vi "ExSubtract2DataFiles.vi"() -> ()   [LabVIEW 2010]
panel:
  in  "Output File Type":u32=67371008
  in  "Output File Name":path
  in  "Input File 2 Type":u32=67371008
  in  "Input File 2 Operation":u32=6
  in  "Input File 1 Name":path
  in  "Input File 2 Name":path
  in  "Input File 1 Operation":u32=6
  in  "Input File 1 Type":u32=67371008
  out "error out":errorcluster
  in  "error in (no error)":errorcluster
  # "ExSubtract2DataFiles.vi\nThis VI will open the both input files, subtract File 2 from File 1\nand save the result to the output file. \nNote that the full path names must be provided for both input\nfiles and the output file."
  # "TIF   = 67174400\n  SPE = 67371008\n  PMI  = 67436544"
  # "6 = Read Only"
  # "TIF   = 67174400\n  SPE = 67371008\n  PMI  = 67436544"
  # "6 = Read Only"
  # "TIF   = 67174400\n  SPE = 67371008\n  PMI  = 67436544"
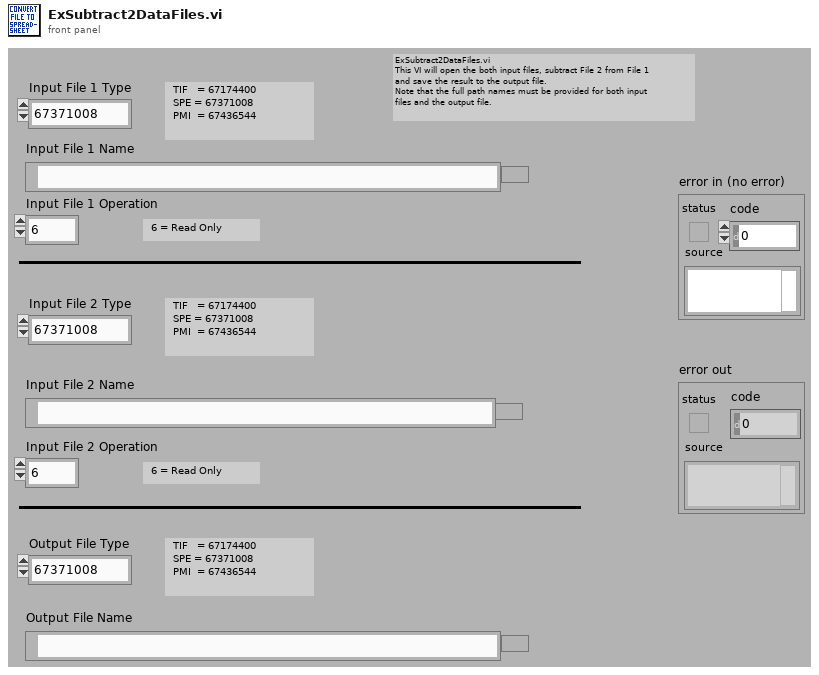
[diagram p1: front panel]
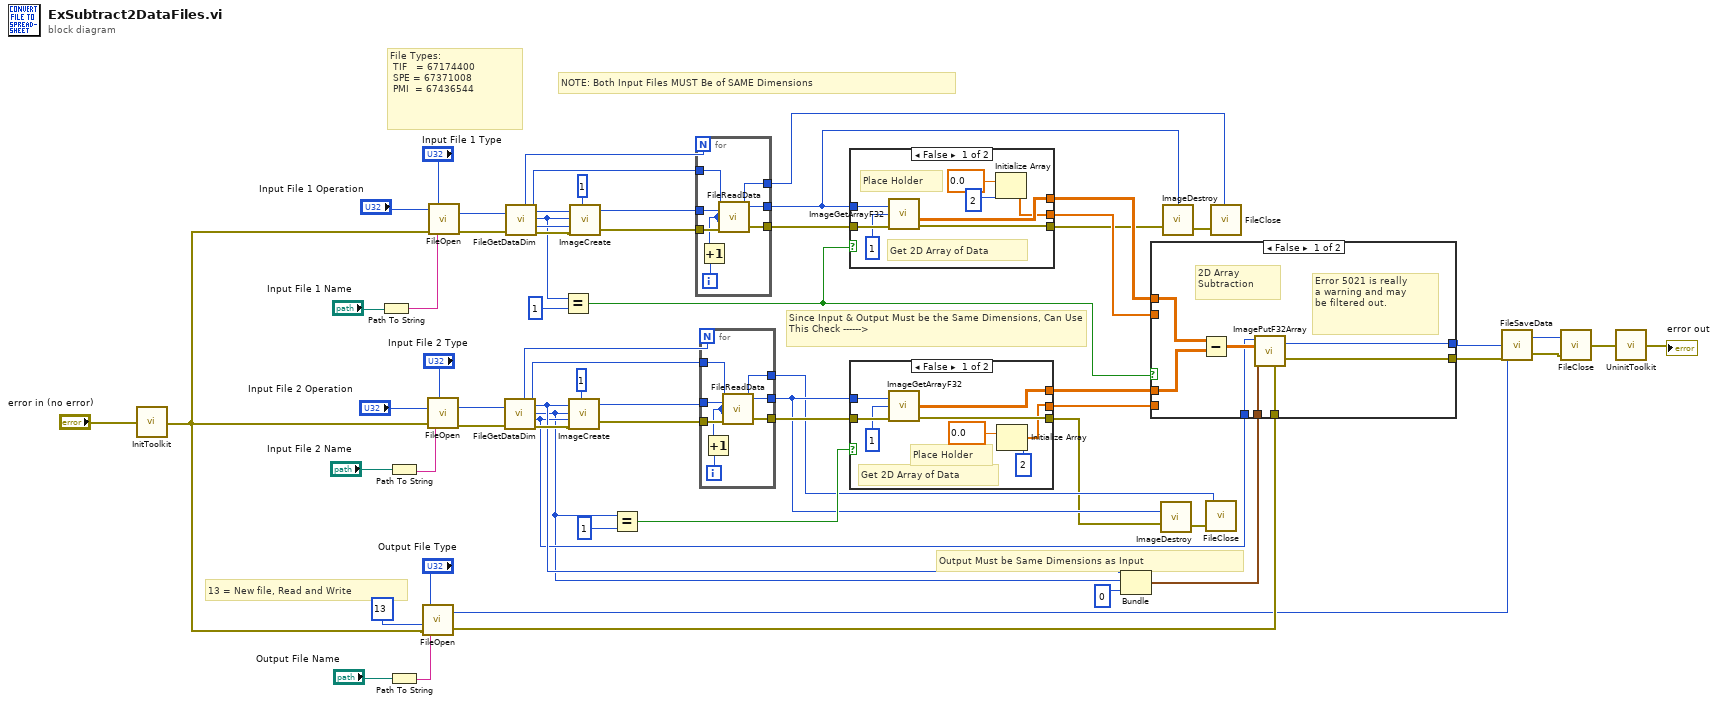
[diagram p0: block diagram]
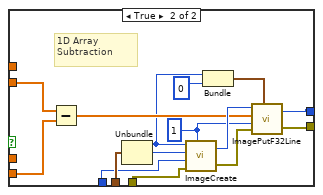
[diagram p2: hidden frame]
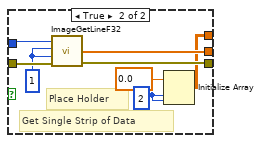
[diagram p3: hidden frame]
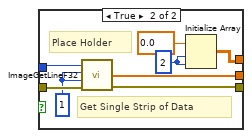
[diagram p4: hidden frame]
diagram:
  # "Since Input & Output Must be the Same Dimensions, Can Use This Check ------>"
  # "NOTE: Both Input Files MUST Be of SAME Dimensions"
  # "Output Must be Same Dimensions as Input"
  # "13 = New file, Read and Write"
  # "File Types:\n TIF   = 67174400\n SPE = 67371008\n PMI  = 67436544"
  n1 = call <userlib>:"InitToolkit.vi"("error in"="error in (no error)") -> ("error out"=w1:errorcluster)
  n2 = Path To String(path="Input File 1 Name") -> (string=w48:string)
  n3 = Path To String(path="Input File 2 Name") -> (string=w37:string)
  n4 = Path To String(path="Output File Name") -> (string=w27:string)
  n5 = call <userlib>:"FileOpen.vi"("error in"=w1, "File Operations"=13, "FileName"=w27, "File Type"="Output File Type") -> ("error out"=w8:errorcluster, "File Handle"=w3:u32)
  n6 = call <userlib>:"FileOpen.vi"("error in"=w1, "File Operations"="Input File 2 Operation", "FileName"=w37, "File Type"="Input File 2 Type") -> ("error out"=w44:errorcluster, "File Handle"=w43:u32)
  n7 = call <userlib>:"FileOpen.vi"("error in"=w1, "File Operations"="Input File 1 Operation", "FileName"=w48, "File Type"="Input File 1 Type") -> ("error out"=w62:errorcluster, "File Handle"=w61:u32)
  n8 = call <userlib>:"FileGetDataDim.vi"("File Handle"=w43, "error in"=w44) -> ("Number of Frames"=w35:u32, "Data Type"=w12:u32, "File Handle"=w34:u32, "X dim"=w13:u32, "Y dim"=w11:u32, "error out"=w42:errorcluster)
  n9 = call <userlib>:"FileGetDataDim.vi"("File Handle"=w61, "error in"=w62) -> ("Number of Frames"=w59:u32, "Data Type"=w26:u32, "File Handle"=w57:u32, "X dim"=w49:u32, "Y dim"=w25:u32, "error out"=w60:errorcluster)
  n10 = Equal?(x=w25, y=1) -> (x = y?=w20:bool)
  n11 = call <userlib>:"ImageCreate.vi"("X dimension"=w13, "Y dimension"=w11, "Data Type"=w12, "error in"=w42, "Number Of Frames"=1) -> ("Image Handle"=w33:u32, "error out"=w32:errorcluster)
  n12 = call <userlib>:"ImageCreate.vi"("X dimension"=w49, "Y dimension"=w25, "Data Type"=w26, "error in"=w60, "Number Of Frames"=1) -> ("Image Handle"=w56:u32, "error out"=w47:errorcluster)
  n13 = Equal?(x=w11, y=1) -> (x = y?=w30:bool)
  n14 = for {
    N: w59 -> [_]
    tunnel: w47 -> [w72]
    tunnel: w57 -> [w71]
    tunnel: w56 -> [w70]
    tunnel: [w65] -> w45
    tunnel: [w67] -> w55
    tunnel: [w66] -> w46
    i -> [w69]
    n15 = Increment(x=w69) -> (x+1=w68:i32)
    n16 = call <userlib>:"FileReadData.vi"("File Handle"=w71, "Start Frame"=w68, "End Frame"=w68, "error in"=w72, "Image Handle"=w70) -> ("File Handle"=w67:u32, "Image Handle"=w66:u32, "error out"=w65:errorcluster)
  }
  n17 = for {
    N: w35 -> [_]
    tunnel: w32 -> [w80]
    tunnel: w34 -> [w79]
    tunnel: w33 -> [w78]
    tunnel: [w73] -> w31
    tunnel: [w75] -> w21
    tunnel: [w74] -> w22
    i -> [w77]
    n18 = Increment(x=w77) -> (x+1=w76:i32)
    n19 = call <userlib>:"FileReadData.vi"("File Handle"=w79, "Start Frame"=w76, "End Frame"=w76, "error in"=w80, "Image Handle"=w78) -> ("File Handle"=w75:u32, "Image Handle"=w74:u32, "error out"=w73:errorcluster)
  }
  n20 = case shown="False" w20 {
    tunnel: w45 -> [w88 w95]
    tunnel: [w86 w96] -> w14
    tunnel: w46 -> [w85 w94]
    tunnel: [w81 w92] -> w17
    tunnel: [w84 w90] -> w19
    frame False {
      # "Place Holder"
      # "Get 2D Array of Data"
      n21 = call <userlib>:"ImageGetArrayF32.vi"("error in"=w88, "Z position"=1, "Image Handle"=w85) -> ("error out"=w86:errorcluster, "Array Float 32"=w84:sgl[][])  [unwired: 1 out]
      n22 = Initialize Array(sgl 0.0, 2) -> (w81:sgl[])
    }
    frame True {
      w89 = 2
      w93 = 1
      # "Place Holder"
      # "Get Single Strip of Data"
      n23 = call <userlib>:"ImageGetLineF32.vi"("error in"=w95, "Z Position"=w93, "Y Position"=w93, "Data Handle"=w94) -> ("error out"=w96:errorcluster, "Array F32"=w92:sgl[])  [unwired: 1 out]
      n24 = Initialize Array(sgl 0.0, w89, w89) -> (w90:sgl[][])
    }
  }
  n25 = case shown="False" w30 {
    tunnel: w31 -> [w104 w111]
    tunnel: [w102 w112] -> w15
    tunnel: w22 -> [w101 w110]
    tunnel: [w97 w108] -> w16
    tunnel: [w100 w105] -> w18
    frame False {
      # "Place Holder"
      # "Get 2D Array of Data"
      n26 = call <userlib>:"ImageGetArrayF32.vi"("error in"=w104, "Z position"=1, "Image Handle"=w101) -> ("error out"=w102:errorcluster, "Array Float 32"=w100:sgl[][])  [unwired: 1 out]
      n27 = Initialize Array(sgl 0.0, 2) -> (w97:sgl[])
    }
    frame True {
      w106 = 2
      w109 = 1
      # "Place Holder"
      # "Get Single Strip of Data"
      n28 = call <userlib>:"ImageGetLineF32.vi"("error in"=w111, "Z Position"=w109, "Y Position"=w109, "Data Handle"=w110) -> ("error out"=w112:errorcluster, "Array F32"=w108:sgl[])  [unwired: 1 out]
      n29 = Initialize Array(sgl 0.0, w106, w106) -> (w105:sgl[][])
    }
  }
  n30 = Bundle("X dim"=w13, "Y dim"=w11, 0) -> (w9:cluster{"X dim":u32, "Y dim":u32, i32})  [unwired: 1 in]
  n31 = case shown="False" w20 {
    tunnel: w19 -> [w119 _]
    tunnel: w18 -> [w120 _]
    tunnel: w17 -> [_ w135]
    tunnel: w16 -> [_ w134]
    tunnel: w12 -> [w117 w131]
    tunnel: w9 -> [w116 w133]
    tunnel: w8 -> [w115 w130]
    tunnel: [w114 w121] -> w6
    tunnel: [w113 w122] -> w7
    frame False {
      # "Error 5021 is really\na warning and may\nbe filtered out."
      # "2D Array Subtraction"
      n32 = Subtract(x=w119, y=w120) -> (x-y=w118:sgl[][])
      n33 = call <userlib>:"ImagePutF32Array.vi"("error in (no error)"=w115, "Image dimensions"=w116, "Image Data"=w118, "Data Type to store as"=w117) -> ("error out"=w114:errorcluster, "Image Handle"=w113:u32)
    }
    frame True {
      w126 = 1
      # "1D Array Subtraction"
      n34 = Subtract(x=w135, y=w134) -> (x-y=w127:sgl[])
      n35 = Unbundle(w133) -> ("X dim"=w125:u32, "Y dim"=w132:u32)  [unwired: 1 out]
      n36 = call <userlib>:"ImageCreate.vi"("X dimension"=w125, "Y dimension"=w132, "Data Type"=w131, "error in"=w130, "Number Of Frames"=w126) -> ("Image Handle"=w129:u32, "error out"=w128:errorcluster)
      n37 = Bundle("X dim"=w125, 0) -> (w123:cluster{"X dim":u32, i32})  [unwired: 1 in]
      n38 = call <userlib>:"ImagePutF32Line.vi"("Image Handle"=w129, "Image Data"=w127, "Y Position"=w126, "error in (no error)"=w128, "Image dimensions"=w123) -> ("Image Handle"=w122:u32, "error out"=w121:errorcluster)
    }
  }
  n39 = call <userlib>:"ImageDestroy.vi"("error in"=w15, "Data handle"=w22) -> ("error out"=w29:errorcluster)
  n40 = call <userlib>:"ImageDestroy.vi"("error in"=w14, "Data handle"=w46) -> ("error out"=w54:errorcluster)
  n41 = call <userlib>:"FileClose.vi"("error in"=w29, "File Handle"=w21) -> ()  [unwired: 1 out]
  n42 = call <userlib>:"FileClose.vi"("error in"=w54, "File Handle"=w55) -> ()  [unwired: 1 out]
  n43 = call <userlib>:"FileSaveData.vi"("error in"=w6, "Image Handle"=w7, "File Handle"=w3) -> ("error out"=w5:errorcluster, "File Handle"=w4:u32)
  n44 = call <userlib>:"FileClose.vi"("error in"=w5, "File Handle"=w4) -> ("error out"=w2:errorcluster)
  n45 = call <userlib>:"UninitToolkit.vi"("error in"=w2) -> ("error out"=→"error out":errorcluster)
